vi "Host_9.vi"() -> ()   [LabVIEW 2020]
panel:
  in  "stop":bool
  out "Dane":waveform(dbl)(graph)
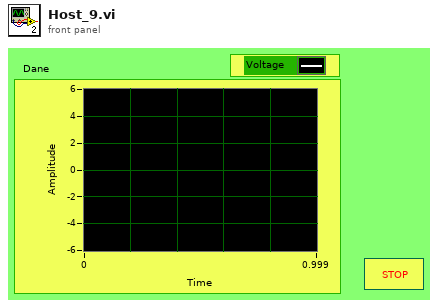
[diagram p1: front panel]
types:
  T1 = enum16{"open", "replace", "create", "open or create", "replace or create", "replace or create with confirmation"}
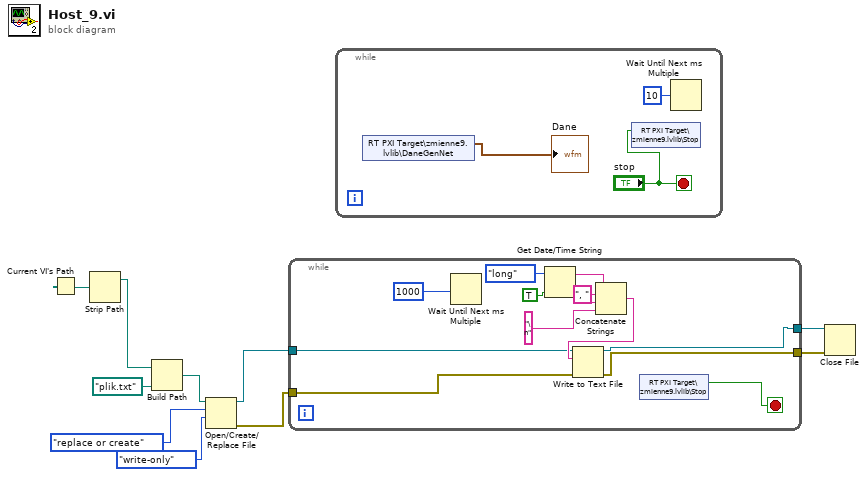
[diagram p0: block diagram]
diagram:
  n1 = Current VI's Path() -> (path=w4:path)
  n2 = Strip Path(path=w4) -> (stripped path=w9:path)  [unwired: 1 out]
  n3 = Build Path(base path=w9, name or relative path=path "plik.txt") -> (appended path=w8:path)
  n4 = Open/Create/Replace File(file path (use dialog)=w8, operation (0:open)=T1."replace or create", access (0:read/write)=enum16{"read/write", "read-only", "write-only"}."write-only") -> (refnum out=w3:refnum<file>, error out=w5:errorcluster)  [unwired: 3 in, 1 out]
  n5 = while {
    tunnel: w5 -> [w18]
    tunnel: w3 -> [w17]
    tunnel: [w16] -> w2
    tunnel: [w15] -> w1
    stop <- w19 stop-if-true
    n6 = Wait Until Next ms Multiple(millisecond multiple=u32 1000 ("milliseconds to wait")) -> ()  [unwired: 1 out]
    n7 = Get Date/Time String(date format (0)=enum16{"short", "long", "abbreviated"}."long", want seconds? (F)=TRUE) -> (date string=w21:string, time string=w12:string)  [unwired: 1 in]
    n8 = Concatenate Strings(w21, ", " ("string"), w12, "\n" ("string")) -> (w20:string)
    n9 = Write to Text File(file (use dialog)=w17, text=w20, error in=w18) -> (refnum out=w15:refnum<file>, error out=w16:errorcluster)  [unwired: 1 in, 1 out]
    n10 = shared-variable "RT PXI Target\\zmienne9.lvlib\\Stop"() -> (w19:bool)  [unwired: 1 in, 1 out]
  }
  n11 = while {
    stop <- "stop" stop-if-true
    n12 = shared-variable "RT PXI Target\\zmienne9.lvlib\\DaneGenNet"() -> (→"Dane":waveform(dbl))  [unwired: 1 in, 1 out]
    n13 = shared-variable "RT PXI Target\\zmienne9.lvlib\\Stop"("stop") -> ()  [unwired: 1 in, 1 out]
    n14 = Wait Until Next ms Multiple(millisecond multiple=u32 10) -> ()  [unwired: 1 out]
  }
  n15 = Close File(refnum=w1, error in=w2) -> ()  [unwired: 2 out]
